vi "Collect Data.vi"(1 "Calibration":T1={"Current Scale Factor kA/V"=1.0, "I->B"=[0.0, 1.0, 0.0], "B->I"=[0.0, 1.0, 0.0]} {"B->I" format="%.5e"; "Current Scale Factor kA/V" format="%.2f"; "I->B" format="%.5e"}, 2 "Scaling Factors":dbl[](array[numeric]) format="%.2f", 5 "Point Number":i32, 6 "stop":bool, 9 "Number to Average":i32=32, 10 "task":refnum<k21>) -> (0 "Output Data":dbl[](array[numeric]) format="%.2e", 4 "Stop":bool)   [LabVIEW 2025]
doc: "Reads the analog inputs, averages the values, reads the GPIB instruments and outputs all the values in a single 1D array.\nScott Hannahs, NHMFL, Sept 1993\nAuthor: Scott Hannahs <sth@magnet.fsu.edu>\n\nThis software is licensed for use under the “MIT License\"\nCopyright (c) 2025 Scott Hannahs, sth@sth@magnet.sthnet.net\n\nPermission is hereby granted, free of charge, to any person obtaining a copy of this software and associated documentation files (the \"Software\"), to deal in the Software without restriction, including without limitation the rights to use, copy, modify, merge, publish, distribute, sublicense, and/or sell copies of the Software, and to permit persons to whom the Software is furnished to do so, subject to the following conditions: The above copyright notice and this permission notice shall be included in all copies or substantial portions of the Software.\n\nTHE SOFTWARE IS PROVIDED \"AS IS\", WITHOUT WARRANTY OF ANY KIND, EXPRESS OR IMPLIED, INCLUDING BUT NOT LIMITED TO THE WARRANTIES OF MERCHANTABILITY, FITNESS FOR A PARTICULAR PURPOSE AND NONINFRINGEMENT. IN NO EVENT SHALL THE AUTHORS OR COPYRIGHT HOLDERS BE LIABLE FOR ANY CLAIM, DAMAGES OR OTHER LIABILITY, WHETHER IN AN ACTION OF CONTRACT, TORT OR OTHERWISE, ARISING FROM, OUT OF OR IN CONNECTION WITH THE SOFTWARE OR THE USE OR OTHER DEALINGS IN THE SOFTWARE."
uses:
  <vilib>/Analysis/baseanly.llb/Mean (DBL).vi
  <vilib>/Analysis/NI_AALBase.lvlib
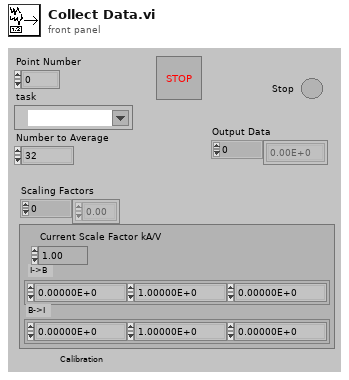
[diagram p1: front panel]
types:
  T1 = cluster{"Current Scale Factor kA/V":dbl, "I->B":dbl[], "B->I":dbl[]}
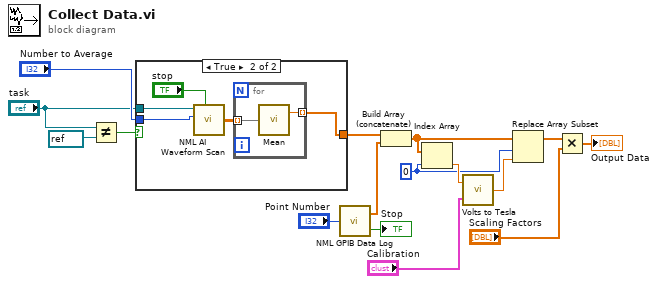
[diagram p0: block diagram]
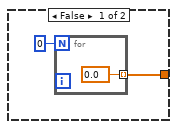
[diagram p2: hidden frame]
diagram:
  w11 = 0
  n1 = Not Equal?(x="task", y=refnum<k21> refnum) -> (x != y?=w15:bool)
  n2 = case shown="True" w15 {
    tunnel: "task" -> [_ w22]
    tunnel: "Number to Average" -> [_ w24]
    tunnel: [w17 w23] -> w6
    frame False {
      n3 = for {
        N: 0 -> [_]
        tunnel: [0.0] -> w17 mode=indexing
      }
    }
    frame True {
      n4 = call "NML AI Waveform Scan.vi"("task/channels in"=w22, "stop"="stop", "Number to Average"=w24) -> ("Scaled data"=w20:dbl[][])  [unwired: 3 in, 2 out]
      n5 = for {
        tunnel: w20 -> [w26] mode=indexing
        tunnel: [w25] -> w23 mode=indexing
        n6 = call-poly <vilib>:"Mean.vi"("X"=w26) -> ("mean"=w25:dbl)  [unwired: 1 out]
      }
    }
  }
  n7 = call "NML GPIB Data Log.vi"("Point #"="Point Number") -> ("GPIB Data"=w2:dbl[], "Stop"=→"Stop":bool)
  n8 = Build Array (concatenate)(w6, w2) -> (w10:dbl[])
  n9 = Index Array(array=w10, index=w11) -> (element=w12:dbl)
  n10 = call "Volts to Tesla.vi"("Calibration"="Calibration", "Console voltage"=w12) -> ("Field"=w13:dbl)
  n11 = Replace Array Subset(array=w10, new element=w13, index=w11) -> (w7:dbl[])
  n12 = Multiply(x=w7, y="Scaling Factors") -> (x*y=→"Output Data":dbl[])
